vi "Get Possible Connections (HW).vi"(8 "error in (no error)":errorcluster, 11 "Routing Channel Ref in":T3 format="%.0x") -> (0 "error out":errorcluster, 2 "Possible Connections":T2(array[cluster]), 3 "Routing Channel Ref out":T3 format="%.0x")   [LabVIEW 2017, in "Routing and Faulting System Explorer.lvlib"]
uses:
  Routing and Faulting System Explorer.lvlib
  <vilib>/NI Veristand/Custom Device API/Custom Device Item Ref.ctl
  Shared/Routing and Faulting Hardware API/Types/Possible Connections for Endpoint.ctl
  <vilib>/NI VeriStand/Custom Device API/Custom Device API.lvlib
  Shared/Routing and Faulting Hardware API/Routing and Faulting Hardware API.lvlib
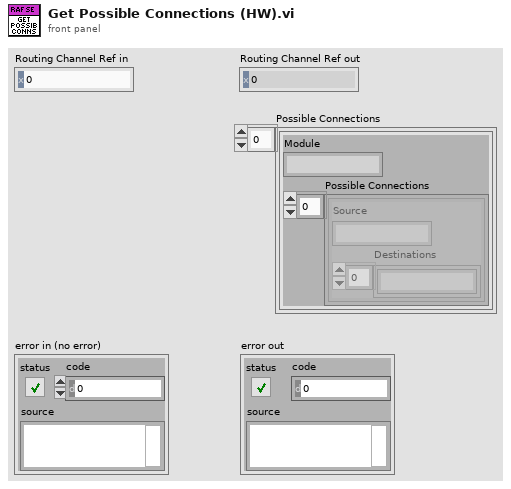
[diagram p1: front panel]
types:
  T1 = typedef "Routing and Faulting Hardware API.lvlib/Possible Connections for Endpoint.ctl" = cluster{"Source":string, "Destinations":string[]}
  T2 = cluster{"Module":string, "Possible Connections":T1[]}[]
  T3 = typedef "Custom Device API.lvlib/Custom Device Item Ref.ctl" = u64
  T4 = cluster{"Formatted Module Path":string, "Possible Connections":T1[]}
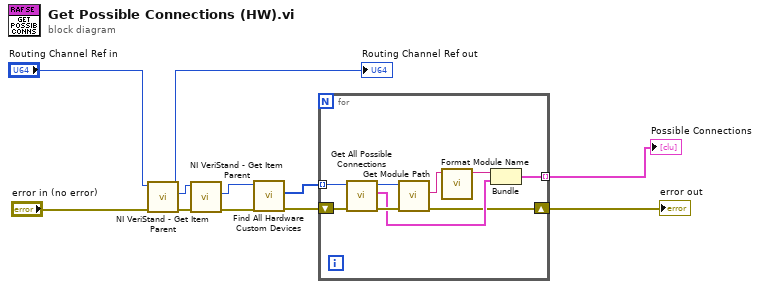
[diagram p0: block diagram]
diagram:
  n1 = call <vilib>:"NI VeriStand - Get Item Parent.vi"("error in (no error)"="error in (no error)", "Item Ref in"="Routing Channel Ref in") -> ("error out"=w9:errorcluster, "Parent Ref"=w10:T3, "Item Ref out"=→"Routing Channel Ref out":T3)  [unwired: 6 in, 1 out]
  n2 = call <vilib>:"NI VeriStand - Get Item Parent.vi"("error in (no error)"=w9, "Item Ref in"=w10) -> ("error out"=w6:errorcluster, "Parent Ref"=w5:T3)  [unwired: 6 in, 2 out]
  n3 = call "Find All Hardware Custom Devices.vi"("error in (no error)"=w6, "Routing and Faulting Ref in"=w5) -> ("error out"=w3:errorcluster, "Hardware Refs"=w4:T3[])  [unwired: 7 in, 1 out]
  n4 = for {
    tunnel: w4 -> [w20] mode=indexing
    shift-right: [w14] -> w1
    shift-left: w3 -> [w19]
    tunnel: [w15] -> w2 mode=indexing
    n5 = call "Get All Possible Connections.vi"("error in (no error)"=w19, "Hardware Ref in"=w20) -> ("error out"=w17:errorcluster, "Possible Connections"=w16:T1[], "Hardware Ref out"=w18:T3)  [unwired: 6 in, 1 out]
    n6 = call "Get Module Path.vi"("error in (no error)"=w17, "Hardware Ref in"=w18) -> ("error out"=w14:errorcluster, "Resource"=w13:string)  [unwired: 6 in, 2 out]
    n7 = call "Format Module Name.vi"("Module Path"=w13) -> ("Formatted Module Path"=w12:string)  [unwired: 10 in]
    n8 = Bundle("Formatted Module Path"=w12, "Possible Connections"=w16) -> (w15:T4)  [unwired: 1 in]
  }
  "error out" <- w1
  "Possible Connections" <- w2
